vi "Input_Commands_Turret.vi"(11 "All Joysticks":T2) -> (3 "Turret Command Inputs":T1)   [LabVIEW 2012]
uses:
  Input_All_Joysticks.ctl
  Input_Single_Joystick.ctl
  <vilib>/Rock Robotics/WPI/Joystick/WPI_JoystickButtonState.ctl
  Inputs_Commands_Turret.ctl
panel:
  in  "Scaling Factor":dbl=1.0
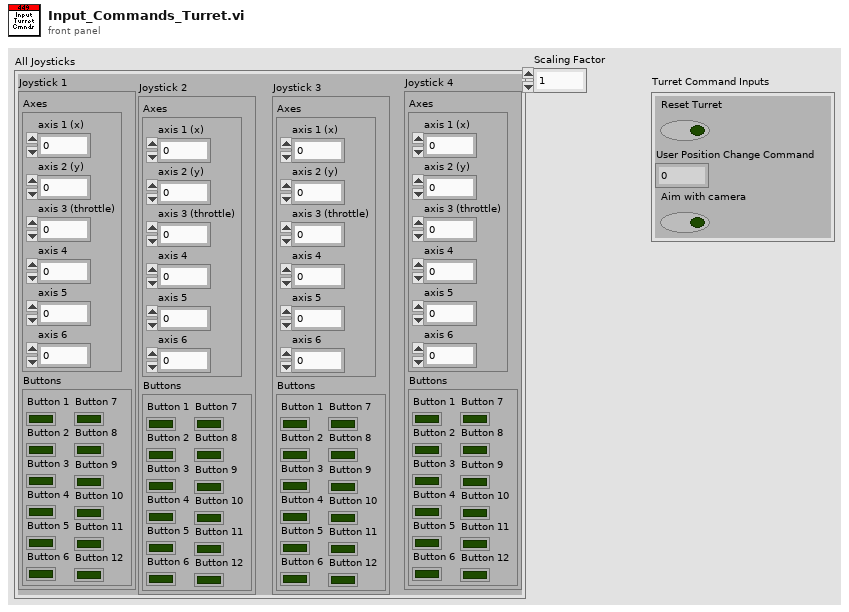
[diagram p1: front panel]
types:
  T1 = typedef "Inputs_Commands_Turret.ctl" = cluster{"Reset Turret":bool, "User Position Change Command":dbl, "Aim with camera":bool}
  T2 = typedef "Input_All_Joysticks.ctl" = cluster{"Joystick 1":T3, "Joystick 2":T3, "Joystick 3":T3, "Joystick 4":T3}
  T3 = typedef "Input_Single_Joystick.ctl" = cluster{"Axes":cluster{"axis 1 (x)":dbl, "axis 2 (y)":dbl, "axis 3 (throttle)":dbl, "axis 4":dbl, "axis 5":dbl, "axis 6":dbl}, "Buttons":T4}
  T4 = typedef "WPI_JoystickButtonState.ctl" = cluster{"Button 1":bool, "Button 2":bool, "Button 3":bool, "Button 4":bool, "Button 5":bool, "Button 6":bool, "Button 7":bool, "Button 8":bool, "Button 9":bool, "Button 10":bool, "Button 11":bool, "Button 12":bool}
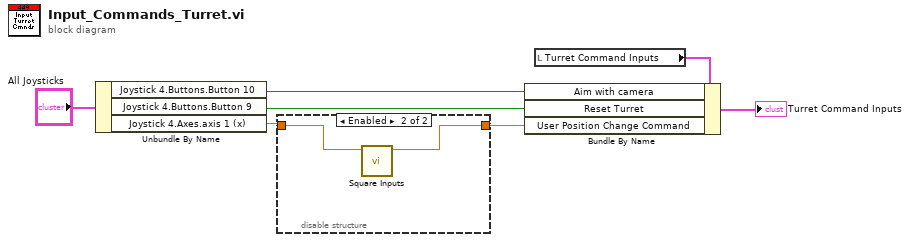
[diagram p0: block diagram]
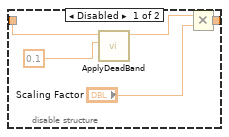
[diagram p2: hidden frame]
diagram:
  n1 = Unbundle By Name("All Joysticks") -> ("Joystick 4.Buttons.Button 10"=w4:bool, "Joystick 4.Buttons.Button 9"=w3:bool, "Joystick 4.Axes.axis 1 (x)"=w6:dbl)
  n2 = disable-structure shown="Enabled" {
    disable-tunnel: w6 -> [w11 w14]
    disable-tunnel: [w9 w13] -> w2
    frame Disabled {
      n3 = call "ApplyDeadBand.vi"("Deadband"=0.1 ("Threshold"), "Input"=w11) -> ("Input with deadband"=w10:dbl)  [unwired: 9 in]
      n4 = Multiply(x=w10, y="Scaling Factor") -> (x*y=w9:dbl)
    }
    frame Enabled {
      n5 = call "Square Inputs.vi"("Input"=w14) -> ("Squared Value"=w13:dbl)  [unwired: 10 in]
    }
  }
  n6 = local read "Turret Command Inputs"() -> (w5:T1)
  n7 = Bundle By Name(cluster=w5, "Aim with camera"=w4, "Reset Turret"=w3, "User Position Change Command"=w2) -> (→"Turret Command Inputs":T1)
